vi "Tell Parent.vi"(4 "Priority":bool, 10 "Msg":refnum<class "Msg.lvclass">, 11 "Base Actor in":refnum<class "Base Actor.lvclass">) -> (0 "Error out":errorcluster)   [LabVIEW 2025, in "jettl.lvlib" / "Actor.lvlib" / "Base Actor.lvclass"]
uses:
  Base Actor.lvclass
  Base Actor.lvclass/Base Actor.ctl
  Relation.ctl
  Actor.lvlib
  Attributes/Attributes/Attributes.lvclass
  Error/Error.lvlib
  Msg/Msg.lvclass
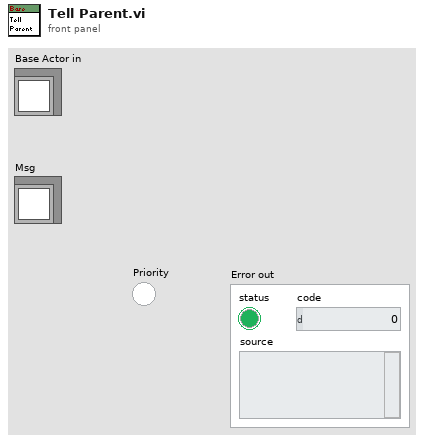
[diagram p1: front panel]
types:
  T1 = typedef "jettl.lvlib/Actor.lvlib/Msg Set.ctl" = set{refnum<class "Msg.lvclass">}
  T2 = typedef "jettl.lvlib/Actor.lvlib/Relation.ctl" = enum16{"Self", "Creator", "Created"}
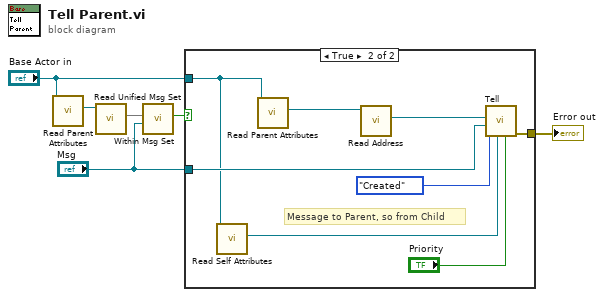
[diagram p0: block diagram]
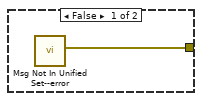
[diagram p2: hidden frame]
diagram:
  n1 = call-dynamic "Read Parent Attributes.vi"("Base Actor in"="Base Actor in") -> ("Parent Attributes"=w3:refnum<class "Attributes.lvclass">)  [unwired: 10 in]
  n2 = call-dynamic "Read Unified Msg Set.vi"("Attributes in"=w3) -> ("Unified Msg Set"=w4:T1)  [unwired: 10 in]
  n3 = call "Within Msg Set.vi"("Msg"="Msg", "Msg Set"=w4) -> ("Within Msg Set"=w6:bool)  [unwired: 9 in]
  n4 = case shown="True" w6 {
    tunnel: "Base Actor in" -> [_ w11]
    tunnel: "Msg" -> [_ w13]
    tunnel: [w7 w10] -> w1
    frame False {
      n5 = call "Msg Not In Unified Set--error.vi"() -> ("Error"=w7:errorcluster)  [unwired: 11 in]
    }
    frame True {
      # "Message to Parent, so from Child"
      n6 = call-dynamic "Read Self Attributes.vi"("Base Actor in"=w11) -> ("Self Attributes"=w14:refnum<class "Attributes.lvclass">)  [unwired: 10 in]
      n7 = call-dynamic "Read Parent Attributes.vi"("Base Actor in"=w11) -> ("Parent Attributes"=w9:refnum<class "Attributes.lvclass">)  [unwired: 10 in]
      n8 = call-dynamic "Read Address.vi"("Attributes in"=w9) -> ("Address"=w8:refnum<user-event>)  [unwired: 10 in]
      n9 = call "Tell.vi"("Priority"="Priority", "Self Attributes"=w14, "Relation"=Relation."Created", "Msg"=w13, "Address"=w8) -> ("Error out"=w10:errorcluster)  [unwired: 6 in]
    }
  }
  "Error out" <- w1
